vi "cno_derivatives.vi"(0 "P":dbl[](array[numeric]), 1 "cno data":T1, 5 "SCALE":dbl[](array[numeric]), 9 "OB":dbl[](array[numeric]), 11 "error in (no error)":errorcluster, 12 "user defined functions":T2) -> (4 "A":dbl[][](array[numeric]), 6 "G":dbl[](array[numeric]), 8 "B":dbl[](array[numeric]), 10 "CONSTRAINT":dbl[](array[numeric]), 14 "number of function calls":i32, 15 "error":errorcluster)   [LabVIEW 2020, in "NI_Gmath.lvlib"]
uses:
  NI_Gmath.lvlib
  cno_user defined functions.ctl
  cno_user objective function ref.ctl
  objective function data.ctl
  cno_data.ctl
  fpuIEEE64_finiteDiffConstants.ctl
  A x Vector.vi
  Real Matrix Condition Number.vi
  zeroes_1d.vi
  Create Special Real Matrix.vi
  zeroes_2d.vi
  NI_AALPro.lvlib
  NI_AALBase.lvlib
panel:
  in  "machine eps":dbl=2.22045e-16 format="%#_6e"
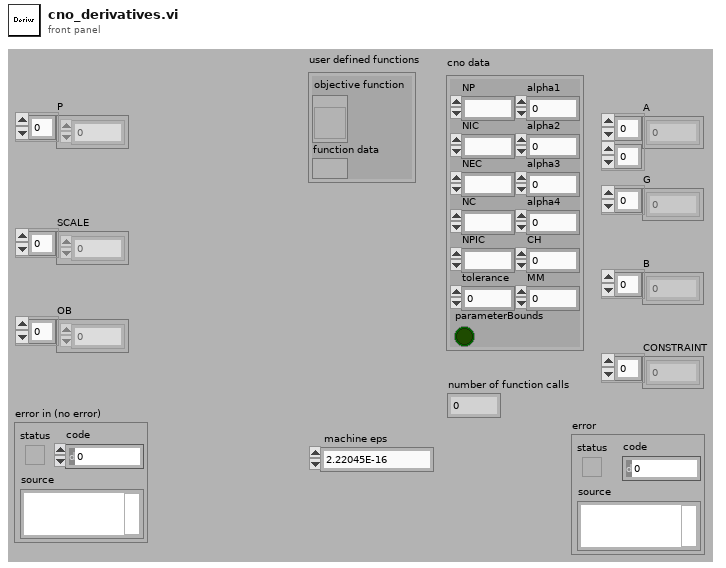
[diagram p1: front panel]
types:
  T1 = typedef "NI_Gmath.lvlib/cno_data.ctl" = cluster{"NP":i32, "NIC":i32, "NEC":i32, "NC":i32, "NPIC":i32, "parameterBounds":bool, "alpha1":dbl, "alpha2":dbl, "alpha3":dbl, "alpha4":dbl, "CH":i32, "MM":i32, "tolerance":dbl}
  T2 = typedef "NI_Gmath.lvlib/cno_user defined functions.ctl" = cluster{"objective function":T3, "function data":T4}
  T3 = typedef "NI_Gmath.lvlib/cno_user objective function ref.ctl" = refnum<vi>
  T4 = typedef "NI_Gmath.lvlib/objective function data.ctl" = variant
  T5 = typedef "NI_Matrix.lvlib/RealMatrix.ctl" = dbl[][]
  T6 = typedef "NI_Gmath.lvlib/fpuIEEE64_finiteDiffConstants.ctl" = dbl
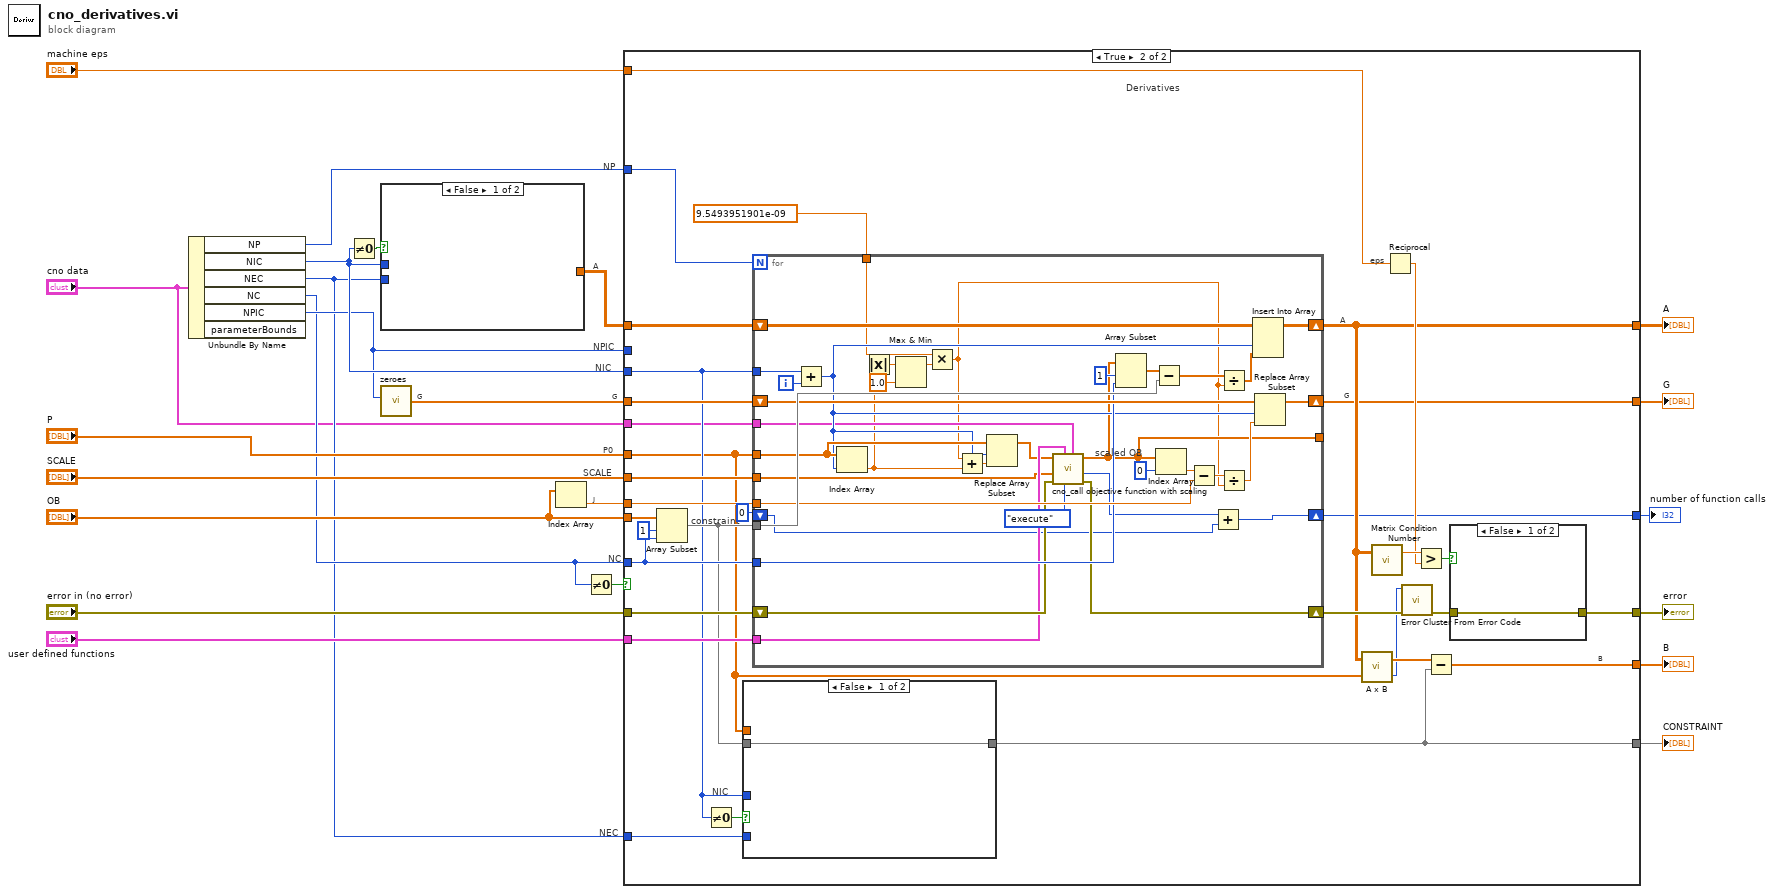
[diagram p0: block diagram]
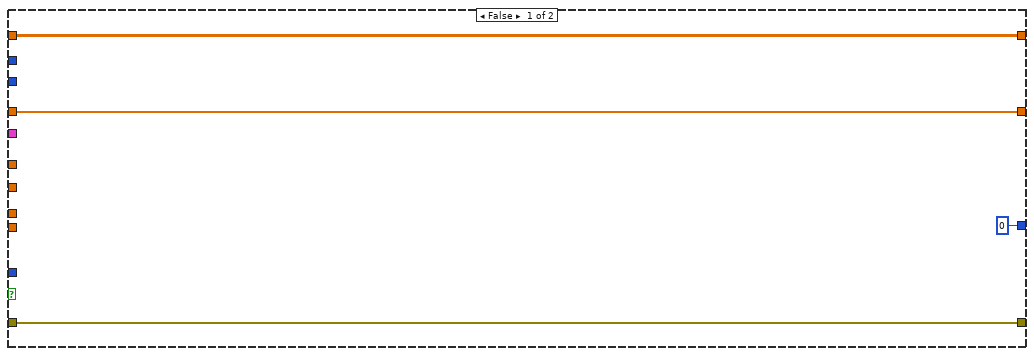
[diagram p2: hidden frame]
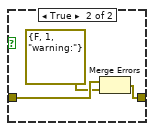
[diagram p3: hidden frame]
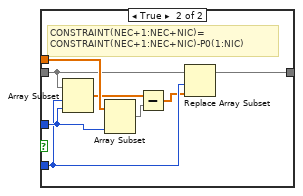
[diagram p4: hidden frame]
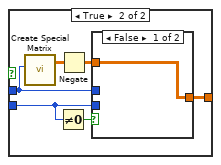
[diagram p5: hidden frame]
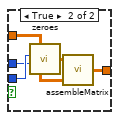
[diagram p6: hidden frame]
diagram:
  # "NP"
  # "NC"
  # "NEC"
  # "G"
  # "SCALE"
  # "P0"
  # "NIC"
  # "NPIC"
  # "J"
  # "G"
  # "A"
  n1 = Unbundle By Name("cno data") -> ("NP"=w16:i32, "NIC"=w15:i32, "NEC"=w4:i32, "NC"=w5:i32, "NPIC"=w14:i32)  [unwired: 1 out]
  n2 = Not Equal To 0?(x=w15) -> (x != 0?=w6:bool)
  n3 = case shown="False" w6 {
    tunnel: w15 -> [_ w25]
    tunnel: w4 -> [_ w26]
    tunnel: [_ w24] -> w10
    frame False {
    }
    frame True {
      n4 = call-poly "Create Special Matrix.vi"("matrix size"=w25) -> ("Special Matrix"=w29:T5)  [unwired: 4 in, 1 out]
      n5 = Not Equal To 0?(x=w26) -> (x != 0?=w28:bool)
      n6 = Negate(x=w29) -> (-x=w27:T5)
      n7 = case shown="False" w28 {
        tunnel: w27 -> [w30 w31]
        tunnel: [w30 w32] -> w24
        tunnel: w26 -> [_ w35]
        tunnel: w25 -> [_ w34]
        frame False {
        }
        frame True {
          n8 = call-poly "zeroes.vi"("m"=w35, "n"=w34) -> ("ones"=w33:dbl[][])  [unwired: 6 in]
          n9 = call "assembleMatrix.vi"("A"=w33, "C"=w31) -> ("ABCD"=w32:dbl[][])  [unwired: 3 in]
        }
      }
    }
  }
  n10 = call-poly "zeroes.vi"("m"=w14) -> ("ones"=w11:dbl[])  [unwired: 7 in]
  n11 = Index Array(array="OB") -> (element=w8:dbl)  [unwired: 1 in]
  n12 = Not Equal To 0?(x=w5) -> (x != 0?=w7:bool)
  n13 = case shown="True" w7 {
    tunnel: w8 -> [_ w63]
    tunnel: "OB" -> [_ w70]
    tunnel: w10 -> [w39 w62]
    tunnel: w11 -> [w38 w64]
    tunnel: w5 -> [_ w65]
    tunnel: "user defined functions" -> [_ w68]
    tunnel: "P" -> [_ w46]
    tunnel: w14 -> [_ _]
    tunnel: w15 -> [_ w58]
    tunnel: w16 -> [_ w67]
    tunnel: "SCALE" -> [_ w66]
    tunnel: w4 -> [_ w59]
    tunnel: "machine eps" -> [_ w57]
    tunnel: "error in (no error)" -> [w37 w71]
    tunnel: [w39 w48] -> w21
    tunnel: [w38 w47] -> w22
    tunnel: [_ w49] -> w23
    tunnel: [w37 w45] -> w20
    tunnel: [_ w44] -> w3
    tunnel: "cno data" -> [_ w43]
    tunnel: [0 w40] -> w1
    frame False {
    }
    frame True {
      w42 = T6 9.5493951901e-09 items=["H_FINITE_DIFF_1"=9.5493951901e-09, "H_FINITE_DIFF_2"=3.2057501263e-06, "H_FINITE_DIFF_4"=0.00033989331283, "H_FINITE_DIFF_K_1"=2.8120287999e-06, "H_FINITE_DIFF_K_2"=9.1341513557e-05, "H_FINITE_DIFF_K_3"=0.00045180790895, "H_FINITE_DIFF_K_4"=0.0014917421406] ("fpuIEEE64")
      # "B"
      # "eps"
      # "A"
      # "G"
      # "NIC"
      # "Derivatives"
      # "constraint"
      n14 = Array Subset(array=w70, index=1, length=w65) -> (w60:dbl[])
      n15 = Not Equal To 0?(x=w58) -> (x != 0?=w61:bool)
      n16 = case shown="False" w61 {
        tunnel: w60 -> [w76 w80]
        tunnel: w59 -> [_ w79]
        tunnel: w58 -> [_ w81]
        tunnel: w46 -> [_ w84]
        tunnel: [w76 w77] -> w44
        frame False {
        }
        frame True {
          # "CONSTRAINT(NEC+1:NEC+NIC)=\nCONSTRAINT(NEC+1:NEC+NIC)-P0(1:NIC)"
          n17 = Array Subset(array=w80, index=w79, length=w81) -> (w83:dbl[])
          n18 = Array Subset(array=w84, length=w81) -> (w82:dbl[])  [unwired: 1 in]
          n19 = Subtract(x=w83, y=w82) -> (x-y=w78:dbl[])
          n20 = Replace Array Subset(array=w80, new element=w78, index=w79) -> (w77:dbl[])
        }
      }
      n21 = for {
        N: w67 -> [_]
        tunnel: w68 -> [w97]
        tunnel: w60 -> [w121]
        tunnel: w46 -> [w118]
        tunnel: w58 -> [w102]
        tunnel: w66 -> [w95]
        tunnel: w65 -> [w109]
        tunnel: w63 -> [w115]
        shift-right: [w111] -> w47
        shift-left: w64 -> [w113]
        shift-right: [w104] -> w48
        shift-left: w62 -> [w110]
        shift-right: [w99] -> w52
        shift-left: w71 -> [w100]
        tunnel: [w98] -> _
        tunnel: w43 -> [w96]
        tunnel: w42 -> [w90]
        shift-right: [w86] -> w40
        shift-left: 0 -> [w85]
        i -> [w120]
        # "scaled OB"
        n22 = Add(x=w102, y=w120) -> (x+y=w103:i32)
        n23 = Index Array(array=w118, index=w103) -> (element=w89:dbl)
        n24 = Absolute Value(x=w89) -> (abs(x)=w91:dbl)
        n25 = Max & Min(x=w91, y=1.0) -> (max(x,y)=w93:dbl)  [unwired: 1 out]
        n26 = Multiply(x=w90, y=w93) -> (x*y=w88:T6)
        n27 = Add(x=w88, y=w89) -> (x+y=w119:T6)
        n28 = Replace Array Subset(array=w118, new element=w119, index=w103) -> (w94:dbl[])
        n29 = call "cno_call objective function with scaling.vi"("cno data"=w96, "function"=enum16{"initialize", "execute"}."execute", "user defined functions"=w97, "error in (no error)"=w100, "scale"=w95, "X"=w94) -> ("error out"=w99:errorcluster, "num function calls"=w87:i32, "out"=w98:dbl[])  [unwired: 3 in]
        n30 = Array Subset(array=w98, index=1, length=w109) -> (w107:dbl[])
        n31 = Subtract(x=w107, y=w121) -> (x-y=w106:dbl[])
        n32 = Index Array(array=w98, index=0) -> (element=w116:dbl)
        n33 = Subtract(x=w116, y=w115) -> (x-y=w114:dbl)
        n34 = Add(x=w87, y=w85) -> (x+y=w86:i32)
        n35 = Divide(x=w106, y=w88) -> (x/y=w105:T6[])
        n36 = Divide(x=w114, y=w88) -> (x/y=w112:T6)
        n37 = Insert Into Array(array=w110, index (col)=w103, new element=w105) -> (w104:T5)  [unwired: 1 in]
        n38 = Replace Array Subset(array=w113, new element=w112, index=w103) -> (w111:dbl[])
      }
      n39 = call-poly "A x B.vi"("Vector"=w46, "A"=w48) -> ("error"=w51:i32, "A x Vector"=w53:dbl[])
      n40 = call-poly "Matrix Condition Number.vi"("Input Matrix"=w48) -> ("condition number"=w56:dbl)  [unwired: 1 in, 1 out]
      n41 = Reciprocal(x=w57) -> (1/x=w55:dbl)
      n42 = call "Error Cluster From Error Code.vi"("error in (no error)"=w52, "error code (0)"=w51) -> ("error out"=w50:errorcluster)  [unwired: 7 in]
      n43 = Greater?(x=w56, y=w55) -> (0:w54:bool)
      n44 = Subtract(x=w53, y=w44) -> (x-y=w49:dbl[])
      n45 = case shown="False" w54 {
        tunnel: w50 -> [w72 w75]
        tunnel: [w72 w73] -> w45
        frame False {
        }
        frame True {
          n46 = Merge Errors(w75, errorcluster {"status"=FALSE, "code"=1, "source"="warning:"} ("error in 2 (no error)")) -> (w73:errorcluster)
        }
      }
    }
  }
  "B" <- w23
  "G" <- w22
  "A" <- w21
  "error" <- w20
  "CONSTRAINT" <- w3
  "number of function calls" <- w1
